vi "Dispose.vi"(8 "error in (no error)":errorcluster, 11 "Room":refnum<class "Room.lvclass">) -> (0 "error out":errorcluster)   [LabVIEW 2020, in "Room.lvclass"]
uses:
  Room.lvclass
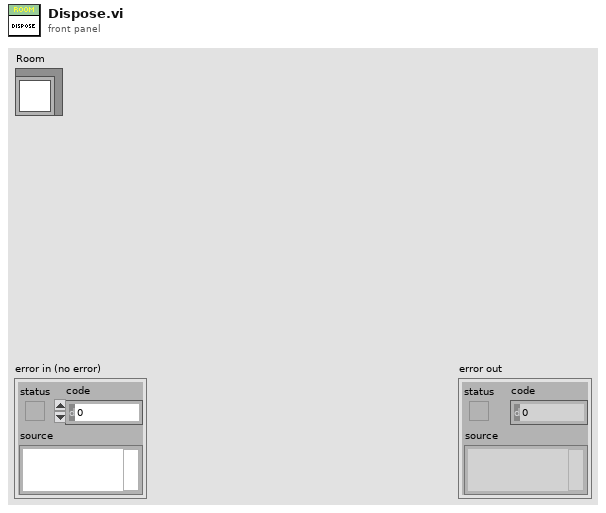
[diagram p1: front panel]
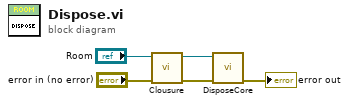
[diagram p0: block diagram]
diagram:
  n1 = call-dynamic "Clousure.vi"("error in (no error)"="error in (no error)", "Room"="Room") -> ("error out"=w1:errorcluster, "Room"=w2:refnum<class "Room.lvclass">)  [unwired: 8 in]
  n2 = call-dynamic "DisposeCore.vi"("error in (no error)"=w1, "Room"=w2) -> ("error out"=→"error out":errorcluster)  [unwired: 8 in, 1 out]
